vi "Check Status.vi"(8 "error in (no error)":errorcluster, 11 "Spectrometer Triax 550 in":refnum<class "Spectrometer Triax 550.lvclass">) -> (0 "error out":errorcluster, 1 "Status":string, 2 "Ready?":bool, 3 "Spectrometer Triax 550 out":refnum<class "Spectrometer Triax 550.lvclass">)   [LabVIEW 2023, in "Spectrometer Triax 550.lvclass"]
doc: "Checks if the instrument is powered on and updates its member data with the instrument's current status."
uses:
  Spectrometer Triax 550.lvclass
  Spectrometer Triax 550.lvclass/Spectrometer Triax 550.ctl
  JY-SPEX-TRIAX/controls.llb/Slits.ctl
  Utility Classes/Scannable/Scannable.lvclass
  JY-SPEX-TRIAX/JY-SPEX-TRIAX.lvlib
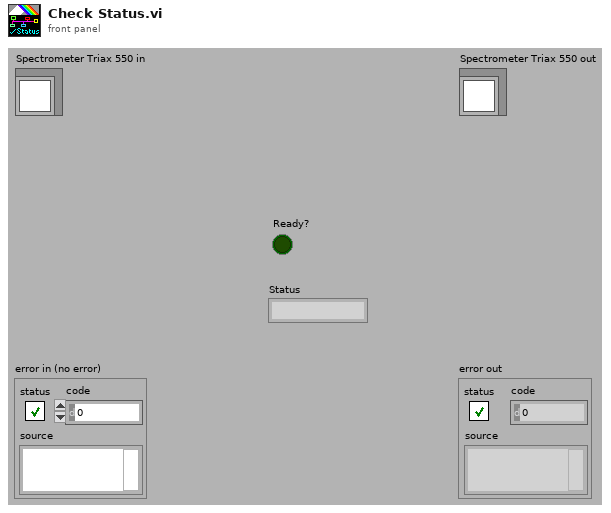
[diagram p1: front panel]
types:
  T1 = typedef "JY-SPEX-TRIAX.lvlib/Slits.ctl" = enum16{"0 (Front/Axial Entrance)", "1 (Side/Lateral Entrance)", "2 (Front/Axial Exit)", "3 (Side/Lateral Exit)"}
  T2 = typedef "JY-SPEX-TRIAX.lvlib/Turret Position (TRIAX).ctl" = enum16{"Grating A", "Grating B", "Grating C"}
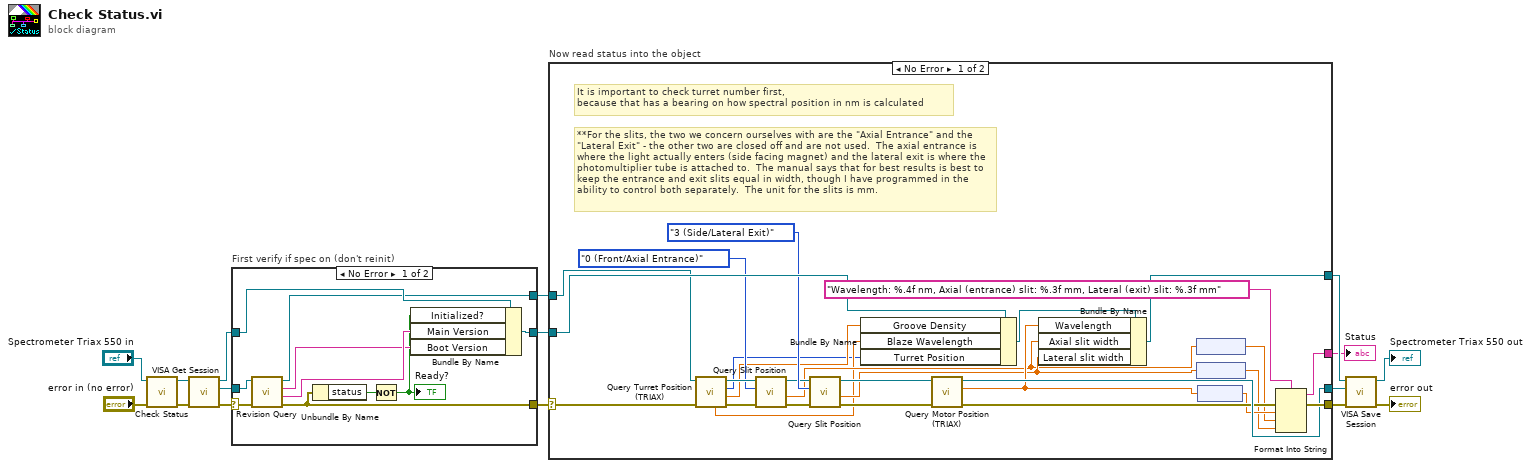
[diagram p0: block diagram]
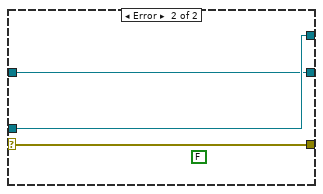
[diagram p2: hidden frame]
diagram:
  n1 = call-parent "Check Status.vi"("error in (no error)"="error in (no error)", "Instrument in"="Spectrometer Triax 550 in") -> ("error out"=w2:errorcluster, "Instrument out"=w14:refnum<class "Spectrometer Triax 550.lvclass">)  [unwired: 8 out]
  n2 = call-dynamic "VISA Get Session.vi"("error in (no error)"=w2, "Instrument.lvclass in"=w14) -> ("error out"=w1:errorcluster, "VISA Resource Name"=w8:refnum<visa-resource-name>, "Instrument.lvclass out"=w10:refnum<class "Spectrometer Triax 550.lvclass">)  [unwired: 7 out]
  n3 = case "First verify if spec on (don't reinit)" shown="No Error" w1 {
    selector: w1 -> [w22 w29]
    tunnel: [w26 w27] -> w11
    tunnel: w10 -> [w25 w27]
    tunnel: w8 -> [w24 w28]
    tunnel: [w23 w29] -> w7
    tunnel: [w20 w28] -> w6
    frame No Error {
      n4 = call "Revision Query.vi"("error in (no error)"=w22, "VISA resource name"=w24) -> ("error out"=w23:errorcluster, "Main Firmware Revision"=w19:string, "Boot Firmware Revision"=w18:string, "VISA resource name out"=w20:refnum<visa-resource-name>)  [unwired: 6 out]
      n5 = Unbundle By Name(w23) -> ("status"=w21:bool)
      n6 = Not(x=w21) -> (.not. x?=w17:bool)
      "Ready?" <- w17
      n7 = Bundle By Name(cluster=w25, "Initialized?"=w17, "Main Version"=w19, "Boot Version"=w18) -> (w26:refnum<class "Spectrometer Triax 550.lvclass">)
    }
    frame Error {
      (unwired) FALSE ("status")
    }
  }
  n8 = case "Now read status into the object" shown="No Error" w7 {
    selector: w7 -> [w36 w58]
    tunnel: w11 -> [w52 w59]
    tunnel: [w51 w59] -> w13
    tunnel: [w54 w58] -> w4
    tunnel: [w53 _] -> w12
    tunnel: w6 -> [w50 w57]
    tunnel: [w41 w57] -> w5
    frame No Error {
      # "**For the slits, the two we concern ourselves with are the \"Axial Entrance\" and the \"Lateral Exit\" - the other two are closed off and are not used.  The axial entrance is where the light actually enters (side facing magnet) and the lateral exit is where the photomultiplier tube is attached to.  The manual says that for best results is best to keep the entrance and exit slits equal in width, though I have programmed in the ability to control both separately.  The unit for the slits is mm."
      # "It is important to check turret number first, \nbecause that has a bearing on how spectral position in nm is calculated"
      n9 = call "Query Turret Position (TRIAX).vi"("error in (no error)"=w36, "VISA resource name"=w50) -> ("error out"=w48:errorcluster, "Groove Density"=w35:dbl[unit], "Turret Position"=w33:T2, "VISA resource name out"=w49:refnum<visa-resource-name>, "Blaze Wavelength"=w34:dbl[unit])  [unwired: 1 in, 4 out]
      n10 = call "Query Slit Position.vi"("error in (no error)"=w48, "Slit (Front/Axial Entrance)"=Slits."0 (Front/Axial Entrance)", "VISA resource name"=w49) -> ("error out"=w45:errorcluster, "Slit Position"=w37:dbl[unit], "VISA resource name out"=w44:refnum<visa-resource-name>)  [unwired: 1 in, 5 out]
      n11 = call "Query Slit Position.vi"("error in (no error)"=w45, "Slit (Front/Axial Entrance)"=Slits."3 (Side/Lateral Exit)", "VISA resource name"=w44) -> ("error out"=w42:errorcluster, "Slit Position"=w38:dbl[unit], "VISA resource name out"=w43:refnum<visa-resource-name>)  [unwired: 1 in, 5 out]
      n12 = Bundle By Name(cluster=w52, "Groove Density"=w35, "Blaze Wavelength"=w34, "Turret Position"=w33) -> (w55:refnum<class "Spectrometer Triax 550.lvclass">)
      n13 = call "Query Motor Position (TRIAX).vi"("error in (no error)"=w42, "VISA resource name"=w43) -> ("error out"=w40:errorcluster, "wavelength"=w39:dbl[unit], "VISA resource name out"=w41:refnum<visa-resource-name>)  [unwired: 1 in, 6 out]
      n14 = Bundle By Name(cluster=w55, "Wavelength"=w39, "Axial slit width"=w37, "Lateral slit width"=w38) -> (w51:refnum<class "Spectrometer Triax 550.lvclass">)
      n15 = node(w37) -> (w31:dbl)
      n16 = node(w38) -> (w30:dbl)
      n17 = node(w39) -> (w32:dbl)
      n18 = Format Into String(format string="Wavelength: %.4f nm, Axial (entrance) slit: %.3f mm, Lateral (exit) slit: %.3f mm", error in=w40, w32, w31, w30) -> (resulting string=w53:string, error out=w54:errorcluster)  [unwired: 1 in]
    }
    frame Error {
    }
  }
  "Status" <- w12
  n19 = call-dynamic "VISA Save Session.vi"("error in (no error)"=w4, "VISA Resource Name"=w5, "Instrument.lvclass in"=w13) -> ("error out"=→"error out":errorcluster, "Instrument.lvclass out"=→"Spectrometer Triax 550 out":refnum<class "Spectrometer Triax 550.lvclass">)  [unwired: 7 out]
